vi "Lezeti_Power_Monitor_11.vi"() -> ()   [LabVIEW 2012]
doc: "This example shows how to use autosetup and acquire a waveform on a single channel."
uses:
  <instrlib>/RIGOL DS1000 Series/Public/Data/Read (Multiple Waveforms).vi
  <vilib>/measure/madcrms.llb/Basic Averaged DC-RMS for 1 Chan.vi
  <vilib>/measure/mascope.llb/Cycle Average and RMS 1 chan.vi
  <vilib>/Utility/file.llb/Write To Spreadsheet File (DBL).vi
  <instrlib>/RIGOL DS1000 Series/RIGOL DS1000 Series.lvlib
  <vilib>/measure/NI_MAPro.lvlib
panel:
  out "Run Date":string
  out "Run Time":string
  out "Elapsed Time (s)":dbl
  in  "Output File":path
  out "Average Power (Watts)":dbl
  out "Instant Power Waveform":waveform(dbl)(graph)
  out "IRMS":dbl
  out "Current Waveform":waveform(dbl)(graph)
  out "VRMS":dbl
  in  "Stop":bool
  out "Voltage Waveform":waveform(dbl)(graph)
  in  "VISA resource name":refnum<visa-resource-name>
  # "For Lezeti Air Conditioning System (Greenpath Tech)\nBy Matsu Thornton\nJuly 2016"
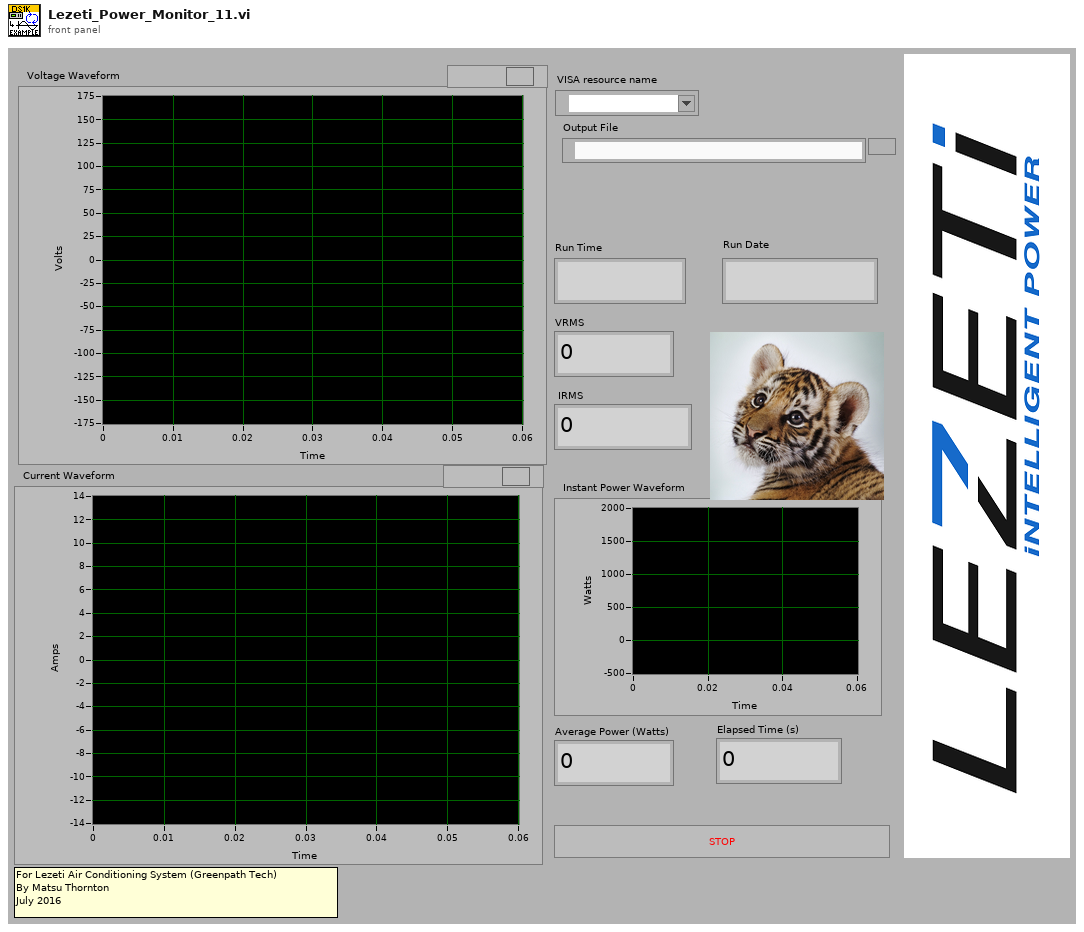
[diagram p1: front panel]
types:
  T1 = typedef "NI_Matrix.lvlib/RealMatrix.ctl" = dbl[][]
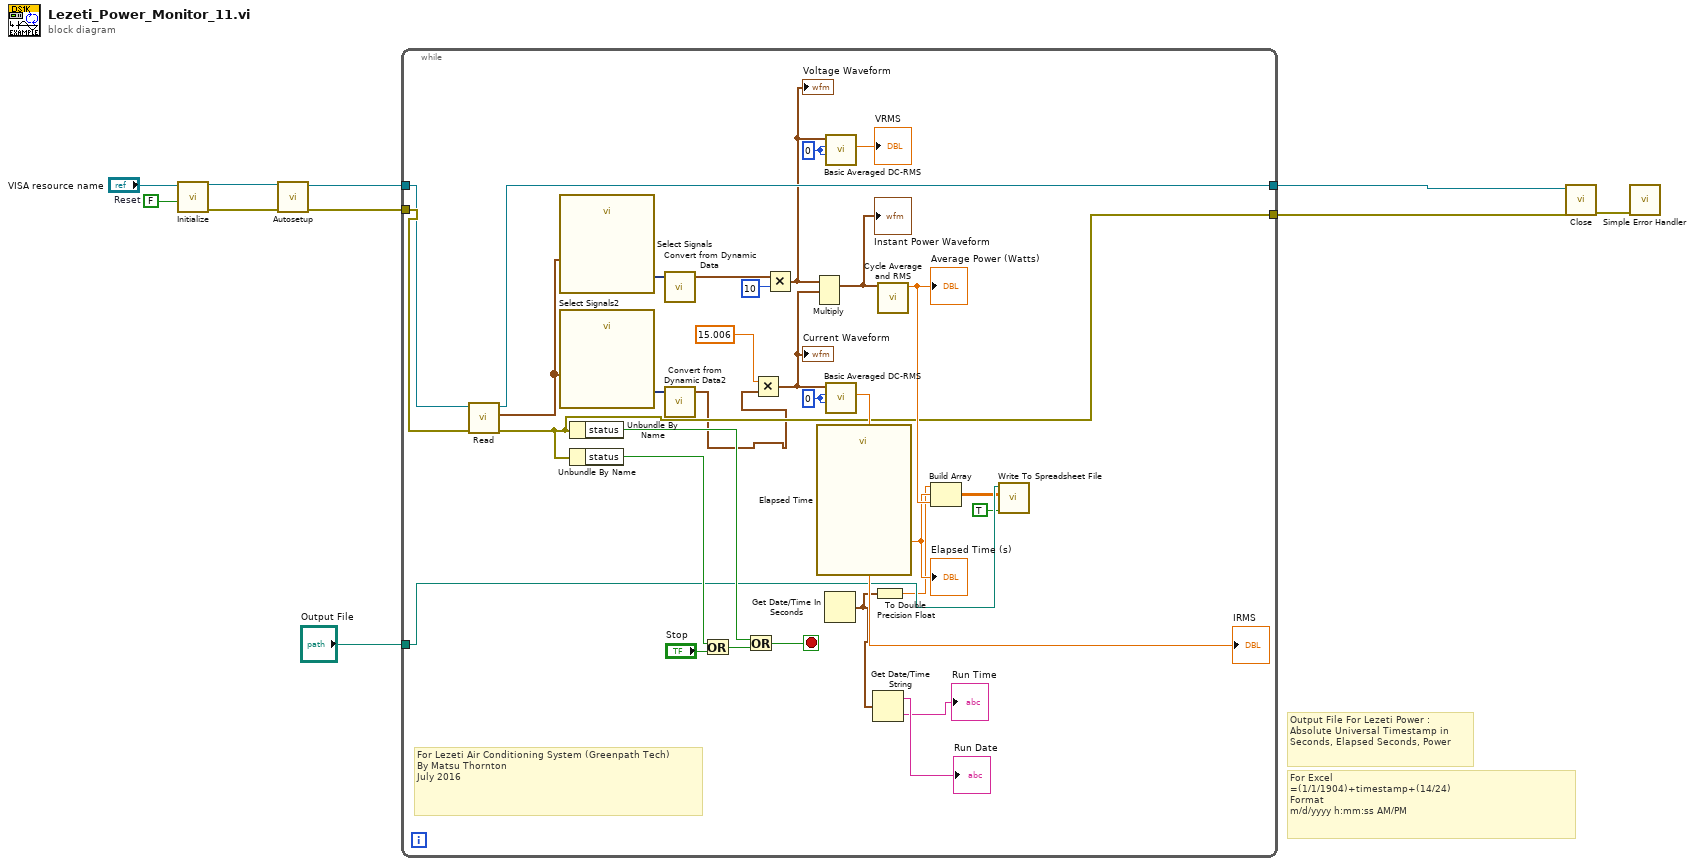
[diagram p0: block diagram]
diagram:
  w3 = FALSE  # Reset
  # "For Excel\n=(1/1/1904)+timestamp+(14/24)\nFormat\nm/d/yyyy h:mm:ss AM/PM"
  # "Output File For Lezeti Power :\nAbsolute Universal Timestamp in Seconds, Elapsed Seconds, Power"
  n1 = call <instrlib>:"Initialize.vi"("Reset (True)"=w3, "VISA resource name"="VISA resource name") -> ("error out"=w7:errorcluster, "VISA resource name out"=w6:refnum<visa-resource-name>)  [unwired: 2 in, 6 out]
  n2 = call <instrlib>:"Autosetup.vi"("error in (no error)"=w7, "VISA resource name"=w6) -> ("error out"=w4:errorcluster, "VISA resource name out"=w5:refnum<visa-resource-name>)  [unwired: 8 out]
  n3 = while {
    tunnel: w5 -> [w19]
    tunnel: w4 -> [w42]
    tunnel: [w41] -> w9
    tunnel: [w20] -> w2
    tunnel: "Output File" -> [w26]
    stop <- w28 stop-if-true
    w36 = 0
    w38 = 0
    # "For Lezeti Air Conditioning System (Greenpath Tech)\nBy Matsu Thornton\nJuly 2016"
    n4 = call-poly <instrlib>:"Read.vi"("error in (no error)"=w42, "VISA resource name"=w19) -> ("error out"=w20:errorcluster, "Waveform Data"=w15:waveform(dbl)[], "VISA resource name out"=w41:refnum<visa-resource-name>)  [unwired: 2 in, 5 out]
    n5 = call "Select Signals"("Signals"=w15) -> ("Signal Out"=w18:dynamicdata)  [unwired: 9 in, 1 out]
    n6 = call "Select Signals2"("Signals"=w15) -> ("Signal Out"=w16:dynamicdata)  [unwired: 9 in, 1 out]
    n7 = Unbundle By Name(w20) -> ("status"=w37:bool)
    n8 = Unbundle By Name(w20) -> ("status"=w40:bool)
    n9 = call "Convert from Dynamic Data"("Dynamic Data Type"=w18) -> ("Waveform"=w17:waveform(dbl))  [unwired: 3 in]
    n10 = call "Convert from Dynamic Data2"("Dynamic Data Type"=w16) -> ("Waveform"=w14:waveform(dbl))  [unwired: 3 in]
    n11 = Or(x=w40, y="Stop") -> (x .or. y?=w29:bool)
    n12 = Or(x=w37, y=w29) -> (x .or. y?=w28:bool)
    n13 = Multiply(x=15.006, y=w14) -> (x*y=w30:waveform(dbl))
    "Current Waveform" <- w30
    n14 = Multiply(x=w17, y=10) -> (x*y=w34:waveform(dbl))
    "Voltage Waveform" <- w34
    n15 = Multiply(1:w30, 2:w34) -> (0:w27:waveform(dbl))  [unwired: 1 in, 1 out]
    "Instant Power Waveform" <- w27
    n16 = call "Elapsed Time"() -> ("Elapsed Time (s)"=w22:dbl)  [unwired: 12 in, 7 out]
    "Elapsed Time (s)" <- w22
    n17 = Get Date/Time In Seconds() -> (seconds since 1Jan1904=w13:timestamp)
    n18 = call-poly <vilib>:"Basic Averaged DC-RMS.vi"("window"=w38, "averaging type"=w38, "signal in"=w34) -> ("RMS value"=→"VRMS":dbl)  [unwired: 5 in, 3 out]
    n19 = call-poly <vilib>:"Basic Averaged DC-RMS.vi"("window"=w36, "averaging type"=w36, "signal in"=w30) -> ("RMS value"=→"IRMS":dbl)  [unwired: 5 in, 3 out]
    n20 = Get Date/Time String(seconds (now)=w13) -> (date string=→"Run Date":string, time string=→"Run Time":string)  [unwired: 2 in]
    n21 = To Double Precision Float(number=w13) -> (double precision float=w21:dbl)
    n22 = call-poly <vilib>:"Cycle Average and RMS.vi"("signal in"=w27) -> ("cycle average"=w23:dbl)  [unwired: 7 in, 3 out]
    "Average Power (Watts)" <- w23
    n23 = Build Array(w21, w22, w23) -> (w24:T1)
    n24 = call-poly <vilib>:"Write To Spreadsheet File.vi"("append to file? (new file:F)"=TRUE, "2D data"=w24, "file path (dialog if empty)"=w26) -> ()  [unwired: 5 in, 1 out]
  }
  n25 = call <instrlib>:"Close.vi"("error in (no error)"=w2, "VISA resource name"=w9) -> ("error out"=w10:errorcluster)  [unwired: 9 out]
  n26 = call <vilib>:"Simple Error Handler.vi"("error in (no error)"=w10) -> ()  [unwired: 1 in, 8 out]
